vi "exel_element.vi"() -> ()   [LabVIEW 2014]
uses:
  <vilib>/addons/_office/NI_ReportGenerationToolkit.lvlib
  <vilib>/Utility/NIReport.llb/NI_report.lvclass
panel:
  in  "border? (F)":bool
  in  "start (-1, -1)":cluster{"row":i32, "column":i32}={"row"=-1, "column"=-1}
  in  "text":string
  in  "report type":T1(ring)
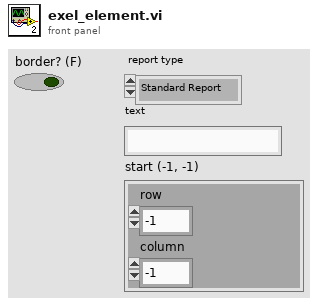
[diagram p1: front panel]
types:
  T1 = enum16{"Standard Report", "HTML", "Word", "Excel"}
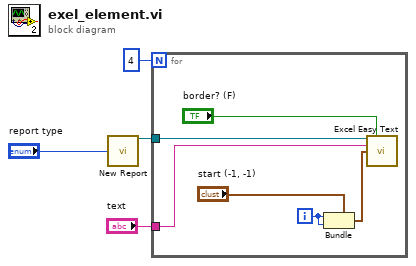
[diagram p0: block diagram]
diagram:
  n1 = call <vilib>:"New Report.vi"("report type"="report type") -> ("report out"=w4:refnum<class "NI_report.lvclass">)  [unwired: 13 in, 1 out]
  n2 = for {
    N: 4 -> [_]
    tunnel: w4 -> [w10]
    tunnel: "text" -> [w9]
    i -> [w6]
    n3 = Bundle(cluster="start (-1, -1)", "row"=w6, "column"=w6) -> (w7:cluster{"row":i32, "column":i32})
    n4 = call <vilib>:"Excel Easy Text.vi"("report in"=w10, "border? (F)"="border? (F)", "text"=w9, "start (-1, -1)"=w7) -> ()  [unwired: 7 in, 5 out]
  }
